vi "EmptyFGVHDTtransfer.vi"(11 "VI in":refnum<vi>) -> ()   [LabVIEW 2016]
uses:
  controls/Enum.ctl
panel:
  out "error out":errorcluster
  in  "error in":errorcluster
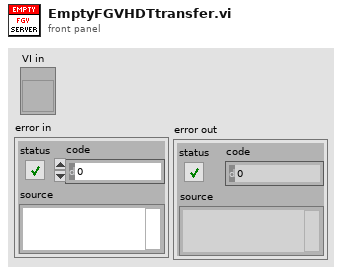
[diagram p1: front panel]
types:
  T1 = typedef "Enum.ctl" = enum16{"Init", "Read", "Write"}
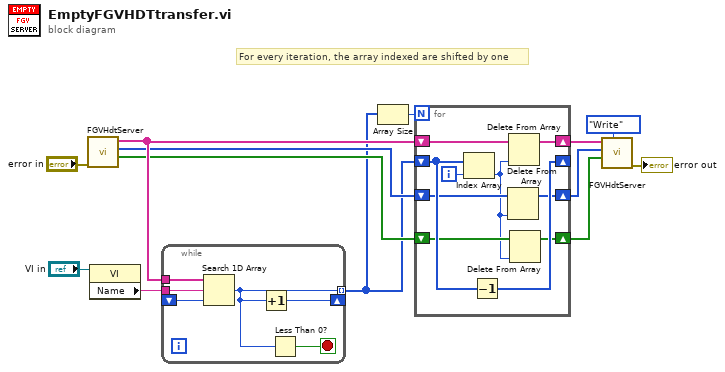
[diagram p0: block diagram]
diagram:
  # "For every iteration, the array indexed are shifted by one"
  n1 = call "FGVHdtServer.vi"("error in"="error in") -> ("UsedOut"=w7:bool[], "HdtTransferSourceOut"=w8:u8[], "OwnerViOut"=w10:string[])  [unwired: 7 in, 1 out]
  n2 = property class="VI"(reference="VI in") -> ("Name"=w11:string)  [unwired: 1 in, 2 out]
  n3 = while {
    tunnel: w11 -> [w19]
    tunnel: w10 -> [w18]
    tunnel: [w16] -> w3 mode=indexing
    shift-right: [w14] -> _
    shift-left: _ -> [w17]
    stop <- w15 stop-if-true
    n4 = Search 1D Array(1D array=w18, element=w19, start index (0)=w17) -> (index of element=w16:i32)
    n5 = Increment(x=w16) -> (x+1=w14:i32)
    n6 = Less Than 0?(x=w16) -> (x < 0?=w15:bool)
  }
  n7 = Array Size(array=w3) -> (size(s)=w4:i32)
  n8 = for {
    N: w4 -> [_]
    shift-right: [w28] -> w9
    shift-left: w10 -> [w29]
    shift-right: [w26] -> _
    shift-left: w3 -> [w27]
    shift-right: [w24] -> w6
    shift-left: w8 -> [w25]
    shift-right: [w21] -> w5
    shift-left: w7 -> [w22]
    i -> [w23]
    n9 = Index Array(array=w27, index=w23) -> (element=w20:i32)
    n10 = Decrement(x=w27) -> (x-1=w26:i32[])
    n11 = Delete From Array(array=w25, index=w20) -> (array with subset deleted=w24:u8[])  [unwired: 1 in, 1 out]
    n12 = Delete From Array(array=w29, index=w20) -> (array with subset deleted=w28:string[])  [unwired: 1 in, 1 out]
    n13 = Delete From Array(array=w22, index=w20) -> (array with subset deleted=w21:bool[])  [unwired: 1 in, 1 out]
  }
  n14 = call "FGVHdtServer.vi"("Enum"=Enum."Write", "UsedIn"=w5, "HDTTransferSourceIn"=w6, "OwnerViIn"=w9) -> ("error out"=→"error out":errorcluster)  [unwired: 4 in, 3 out]
